vi "Script Icon Text.vi"(8 "error in":errorcluster, 9 "VI Refs.Name VI":refnum<vi>, 10 "Name Refs.Name VI":refnum<vi>) -> (0 "error out":errorcluster)   [LabVIEW 2025, in "_Msg Rescript.lvlib" / "_Msg Rescript.lvclass"]
uses:
  _Msg Rescript.lvclass
  _Msg Rescript.lvclass/_Msg Rescript.ctl
  <vilib>/LabVIEW Icon API/lv_icon/Classes/Icon Framework/Icon Framework.lvclass
  <vilib>/LabVIEW Icon API/lv_icon/Classes/Icon/Icon.lvclass
  <vilib>/LabVIEW Icon API/LabVIEW Icon API.lvlib
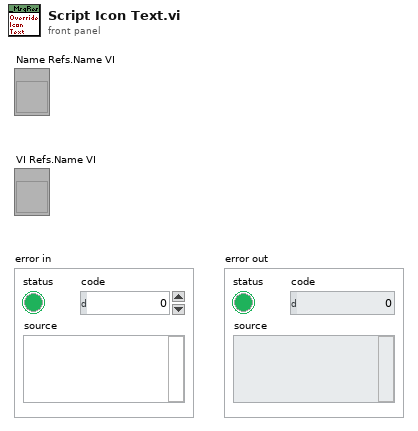
[diagram p1: front panel]
types:
  T1 = typedef "BodyText.ctl" = cluster{"Line 1 text":string, "Line 2 text":string, "Line 3 text":string, "Line 4 text":string, "Line 1 color":u32, "Line 2 color":u32, "Line 3 color":u32, "Line 4 color":u32, "Body Text Spec":cluster{"Font":T2, "Alignment":T3, "Size":u8}, "Center text vertically":bool, "Capitalize Text":bool}
  T2 = typedef "Font.ctl" = string
  T3 = typedef "Alignment.ctl" = u16
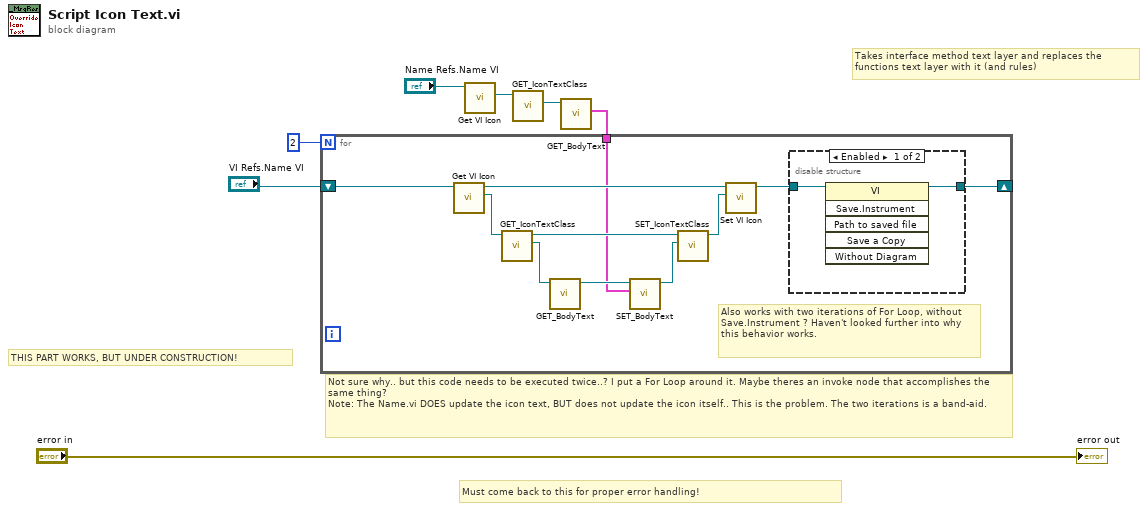
[diagram p0: block diagram]
diagram:
  # "Must come back to this for proper error handling!"
  # "Takes interface method text layer and replaces the functions text layer with it (and rules)"
  # "THIS PART WORKS, BUT UNDER CONSTRUCTION!"
  # "Not sure why.. but this code needs to be executed twice..? I put a For Loop around it. Maybe theres an invoke node that accomplishes the same thing?\nNote: The Name.vi DOES update the icon text, BUT does not update the icon itself.. This is the problem. The two iterations is a band-aid."
  n1 = call <vilib>:"Get VI Icon.vi"("VI Refnum in"="Name Refs.Name VI") -> ("Icon"=w7:refnum<class "Icon.lvclass">)  [unwired: 8 in, 2 out]
  n2 = call-dynamic "GET_IconTextClass.vi"("Icon.lvclass in"=w7) -> ("Icon Framework.lvclass"=w6:refnum<class "Icon Framework.lvclass">)  [unwired: 8 in, 2 out]
  n3 = call-dynamic "GET_BodyText.vi"("Icon Framework.lvclass in"=w6) -> ("Body Text"=w5:T1)  [unwired: 7 in, 3 out]
  n4 = for {
    N: 2 -> [_]
    tunnel: w5 -> [w10]
    shift-right: [w8] -> _
    shift-left: "VI Refs.Name VI" -> [w18]
    # "Also works with two iterations of For Loop, without Save.Instrument ? Haven't looked further into why this behavior works."
    n5 = call <vilib>:"Get VI Icon.vi"("VI Refnum in"=w18) -> ("Icon"=w13:refnum<class "Icon.lvclass">, "VI Refnum out"=w12:refnum<vi>)  [unwired: 8 in, 1 out]
    n6 = call-dynamic "GET_IconTextClass.vi"("Icon.lvclass in"=w13) -> ("Icon Framework.lvclass"=w16:refnum<class "Icon Framework.lvclass">, "Icon.lvclass out"=w15:refnum<class "Icon.lvclass">)  [unwired: 8 in, 1 out]
    n7 = call-dynamic "GET_BodyText.vi"("Icon Framework.lvclass in"=w16) -> ("Icon Framework.lvclass out"=w14:refnum<class "Icon Framework.lvclass">)  [unwired: 7 in, 3 out]
    n8 = call-dynamic "SET_BodyText.vi"("Body Text"=w10, "Icon Framework.lvclass in"=w14) -> ("Icon Framework.lvclass out"=w17:refnum<class "Icon Framework.lvclass">)  [unwired: 8 in, 1 out]
    n9 = call-dynamic "SET_IconTextClass.vi"("Icon Framework.lvclass"=w17, "Icon.lvclass in"=w15) -> ("Icon.lvclass out"=w11:refnum<class "Icon.lvclass">)  [unwired: 8 in, 1 out]
    n10 = call <vilib>:"Set VI Icon.vi"("Icon"=w11, "VI Refnum in"=w12) -> ("VI Refnum out"=w9:refnum<vi>)  [unwired: 8 in, 1 out]
    n11 = disable-structure shown="Enabled" {
      disable-tunnel: w9 -> [w20 w21]
      disable-tunnel: [w19 w21] -> w8
      frame Enabled {
        n12 = invoke class="VI" method="Save.Instrument"(reference=w20) -> (reference out=w19:refnum<vi>)  [unwired: 5 in, 5 out]
      }
      frame Disabled {
      }
    }
  }
  "error out" <- "error in"
